vi "On Acquisition Stop.vi"(8 "error in (no error)":errorcluster, 11 "Camera_Prime95B in":refnum<class "Camera_Prime95B.lvclass">) -> (0 "error out":errorcluster, 3 "Camera_Prime95B out":refnum<class "Camera_Prime95B.lvclass">)   [LabVIEW 2020, in "Camera_Prime95B.lvlib" / "Camera_Prime95B.lvclass"]
uses:
  Camera_Prime95B.lvclass
  E:/Development/DevHardSoftware/MicroscopyFramework/Model/Hardware Layer/Real Hardware/Camera_Prime95B/Camera_Prime95B/Dependencies/PVCamNET.dll
  Dependencies/PVCamNET.dll
  Hardware Abstraction Layer/Component/Device/Device/DeviceStatus.ctl
  Hardware Abstraction Layer/Component/Device/Device/Device.lvlib
  Controls/Camera Status.ctl
  Controls/Wait For Stop Status.ctl
  <vilib>/ActorFramework/Actor/Actor.lvclass
  Interface/DataListener Messages/OnDataChange Msg/OnDataChange Msg.lvclass
  Hardware Abstraction Layer/Component/Device/Device/DataExchange.ctl
  Interface/DataListener/DataListener.lvclass
  C:/Program Files/National Instruments/LabVIEW 2020/vi.lib/ActorFramework/Actor/Actor.lvclass
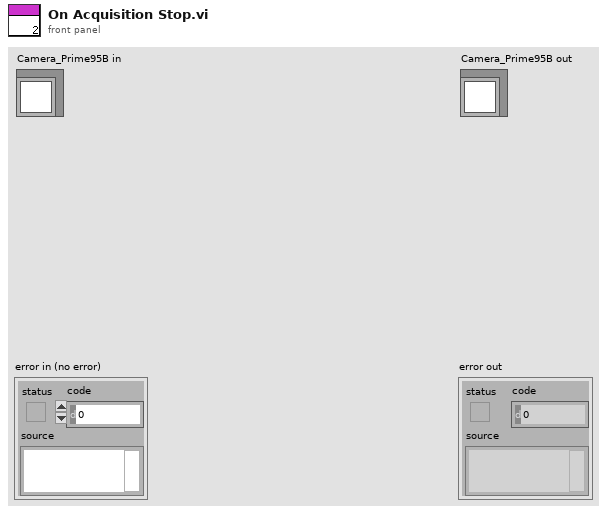
[diagram p1: front panel]
types:
  T1 = typedef "DataListener.lvclass/DataExchange.ctl" = cluster{"Source":string, "Destination":string, "Description":string, "value":variant}
  T2 = typedef "Camera_Prime95B.lvlib/Camera_Prime95B.lvclass/Wait For Stop Status.ctl" = i32
  T3 = typedef "Camera_Prime95B.lvlib/Camera_Prime95B.lvclass/Camera Status.ctl" = i32
  T4 = typedef "Device.lvlib/DeviceStatus.ctl" = i32
  T5 = cluster{"x":dbl, "y":dbl, "width":dbl, "height":dbl}
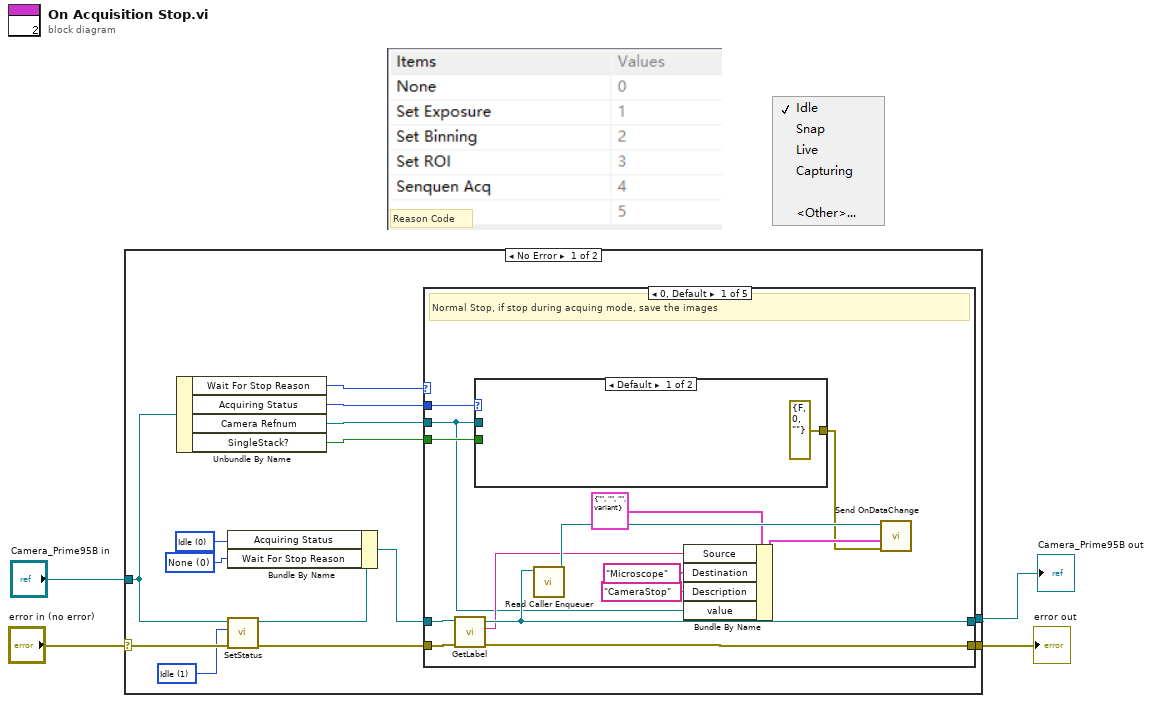
[diagram p0: block diagram]
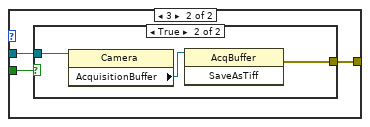
[diagram p2: hidden frame]
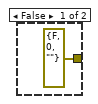
[diagram p3: hidden frame]
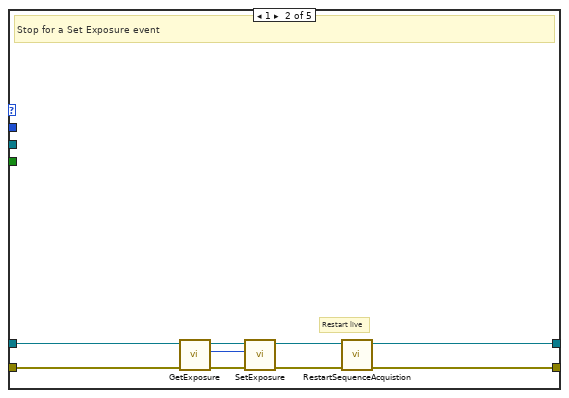
[diagram p4: hidden frame]
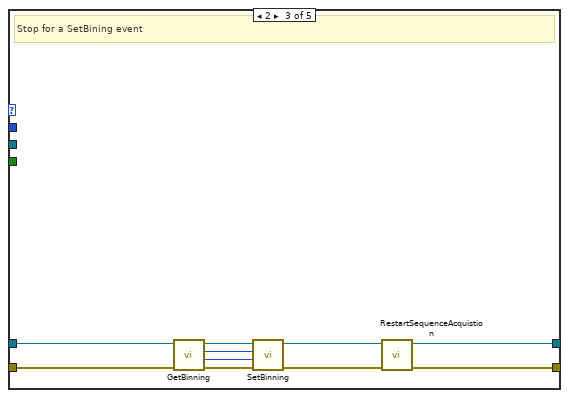
[diagram p5: hidden frame]
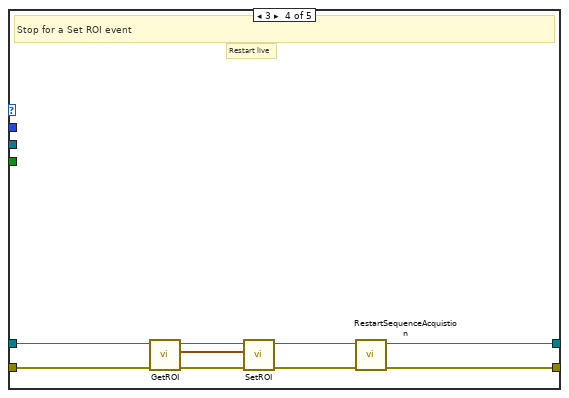
[diagram p6: hidden frame]
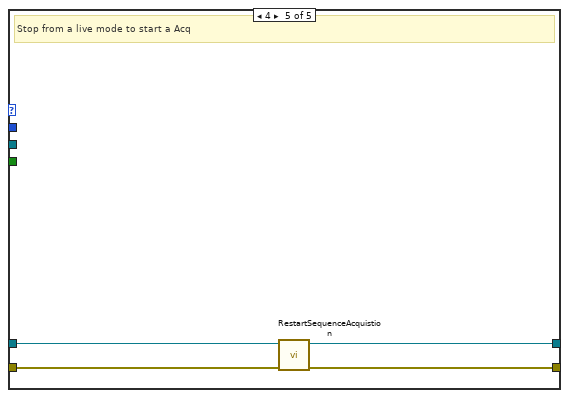
[diagram p7: hidden frame]
diagram:
  # "Reason Code"
  n1 = case shown="No Error" "error in (no error)" {
    selector: "error in (no error)" -> [w13 w74]
    tunnel: [w12 w74] -> w3
    tunnel: [w14 w73] -> w1
    tunnel: "Camera_Prime95B in" -> [w10 w73]
    frame No Error {
      w7 = T2 0 items=["None", "Set Exposure", "Set Binning", "Set ROI", "Sequence Acq", ""] ("Wait For Stop Reason")
      w8 = T3 0 items=["Idle", "Snap", "Live", "Capturing", ""] ("Acquiring Status")
      w9 = T4 1 items=["Offline", "Idle", "Busy"] ("Status")
      n2 = Unbundle By Name(w10) -> ("Wait For Stop Reason"=w18:T2, "Acquiring Status"=w17:T3, "Camera Refnum"=w16:refnum<k24>, "SingleStack?"=w15:bool)
      n3 = call-dynamic "SetStatus.vi"("error in (no error)"=w13, "Status"=w9, "GRMActor in"=w10) -> ("error out"=w11:errorcluster, "GRMActor out"=w6:refnum<class "Camera_Prime95B.lvclass">)  [unwired: 7 in]
      n4 = Bundle By Name(cluster=w6, "Acquiring Status"=w8, "Wait For Stop Reason"=w7) -> (w5:refnum<class "Camera_Prime95B.lvclass">)
      n5 = case shown="0, Default" w18 {
        tunnel: w5 -> [w23 w41 w59 w68 w72]
        tunnel: w17 -> [w32 _ _ _ _]
        tunnel: w16 -> [w20 _ _ _ _]
        tunnel: w15 -> [w31 _ _ _ _]
        tunnel: [w22 w45 w52 w62 w71] -> w14
        tunnel: w11 -> [w30 w44 w51 w61 w70]
        tunnel: [w24 w43 w50 w60 w69] -> w12
        frame 0, Default {
          # "Normal Stop, if stop during acquing mode, save the images"
          n6 = call-dynamic "GetLabel.vi"("error in (no error)"=w30, "GRMActor in"=w23) -> ("error out"=w24:errorcluster, "Label"=w21:string, "GRMActor out"=w22:refnum<class "Camera_Prime95B.lvclass">)  [unwired: 7 in]
          n7 = case shown="Default" w32 {
            tunnel: w20 -> [_ w36]
            tunnel: w31 -> [_ w35]
            tunnel: [errorcluster {"status"=FALSE, "code"=0, "source"=""} ("error out") w34] -> w19
            frame Default {
            }
            frame 3 {
              n8 = case shown="True" w35 {
                tunnel: w36 -> [_ w40]
                tunnel: [errorcluster {"status"=FALSE, "code"=0, "source"=""} ("error out") w38] -> w34
                frame False {
                }
                frame True {
                  n9 = property class="Camera"(reference=w40) -> ("AcquisitionBuffer"=w39:refnum<k24>)  [unwired: 1 in, 2 out]
                  n10 = invoke class="AcqBuffer" method="SaveAsTiff"(reference=w39) -> (error out=w38:errorcluster)  [unwired: 2 in, 2 out]
                }
              }
            }
          }
          n11 = call <vilib>:"Read Caller Enqueuer.vi"("Actor"=w22) -> ("Caller Enqueuer"=w29:refnum<class "Message Enqueuer.lvclass">)  [unwired: 10 in]
          n12 = Bundle By Name(cluster=T1 {"Source"="", "Destination"="", "Description"="", "value"=variant} ("DataExchange"), "Source"=w21, "Destination"="Microscope", "Description"="CameraStop", "value"=w20) -> (w27:T1)
          n13 = call "Send OnDataChange.vi"("error in (no error)"=w19, "DataExchange"=w27, "Message Enqueuer"=w29) -> ()  [unwired: 7 in, 2 out]
        }
        frame 1 {
          # "Restart live"
          # "Stop for a Set Exposure event"
          n14 = call-dynamic "GetExposure.vi"("error in (no error)"=w44, "Camera in"=w41) -> ("error out"=w47:errorcluster, "Setting.Exposure"=w48:i32, "Camera out"=w49:refnum<class "Camera_Prime95B.lvclass">)  [unwired: 7 in]
          n15 = call-dynamic "SetExposure.vi"("error in (no error)"=w47, "Setting.Exposure"=w48, "Camera_Prime95B in"=w49) -> ("error out"=w46:errorcluster, "Camera_Prime95B out"=w42:refnum<class "Camera_Prime95B.lvclass">)  [unwired: 7 in]
          n16 = call-dynamic "RestartSequenceAcquistion.vi"("error in (no error)"=w46, "Camera_Prime95B in"=w42) -> ("error out"=w43:errorcluster, "Camera_Prime95B out"=w45:refnum<class "Camera_Prime95B.lvclass">)  [unwired: 8 in]
        }
        frame 2 {
          # "Stop for a SetBining event"
          n17 = call-dynamic "GetBinning.vi"("error in (no error)"=w51, "Camera in"=w59) -> ("error out"=w55:errorcluster, "Setting.Binning.BinY"=w53:i32, "Setting.Binning.BinX"=w54:i32, "Camera out"=w56:refnum<class "Camera_Prime95B.lvclass">)  [unwired: 6 in]
          n18 = call-dynamic "SetBinning.vi"("error in (no error)"=w55, "Setting.Binning.BinY"=w53, "Setting.Binning.BinX"=w54, "Camera_Prime95B in"=w56) -> ("error out"=w57:errorcluster, "Camera_Prime95B out"=w58:refnum<class "Camera_Prime95B.lvclass">)  [unwired: 6 in]
          n19 = call-dynamic "RestartSequenceAcquistion.vi"("error in (no error)"=w57, "Camera_Prime95B in"=w58) -> ("error out"=w50:errorcluster, "Camera_Prime95B out"=w52:refnum<class "Camera_Prime95B.lvclass">)  [unwired: 8 in]
        }
        frame 3 {
          # "Restart live"
          # "Stop for a Set ROI event"
          n20 = call-dynamic "GetROI.vi"("error in (no error)"=w61, "Camera in"=w68) -> ("error out"=w65:errorcluster, "Setting.ROI"=w64:T5, "Camera out"=w66:refnum<class "Camera_Prime95B.lvclass">)  [unwired: 7 in]
          n21 = call-dynamic "SetROI.vi"("error in (no error)"=w65, "Setting.ROI"=w64, "Camera_Prime95B in"=w66) -> ("error out"=w63:errorcluster, "Camera_Prime95B out"=w67:refnum<class "Camera_Prime95B.lvclass">)  [unwired: 7 in]
          n22 = call-dynamic "RestartSequenceAcquistion.vi"("error in (no error)"=w63, "Camera_Prime95B in"=w67) -> ("error out"=w60:errorcluster, "Camera_Prime95B out"=w62:refnum<class "Camera_Prime95B.lvclass">)  [unwired: 8 in]
        }
        frame 4 {
          # "Stop from a live mode to start a Acq"
          n23 = call-dynamic "RestartSequenceAcquistion.vi"("error in (no error)"=w70, "Camera_Prime95B in"=w72) -> ("error out"=w69:errorcluster, "Camera_Prime95B out"=w71:refnum<class "Camera_Prime95B.lvclass">)  [unwired: 8 in]
        }
      }
    }
    frame Error {
    }
  }
  "error out" <- w3
  "Camera_Prime95B out" <- w1
